vi "val_vagy_vel.vi"(11 "Becenév":string) -> (3 "-val/vel rag":waveform(dbl)[](array[waveform]))   [LabVIEW 2014]
panel:
  out "Boolean":bool
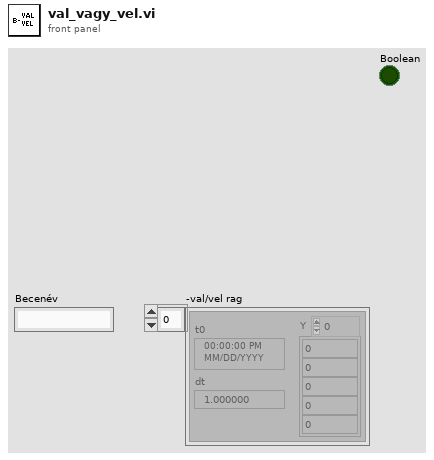
[diagram p1: front panel]
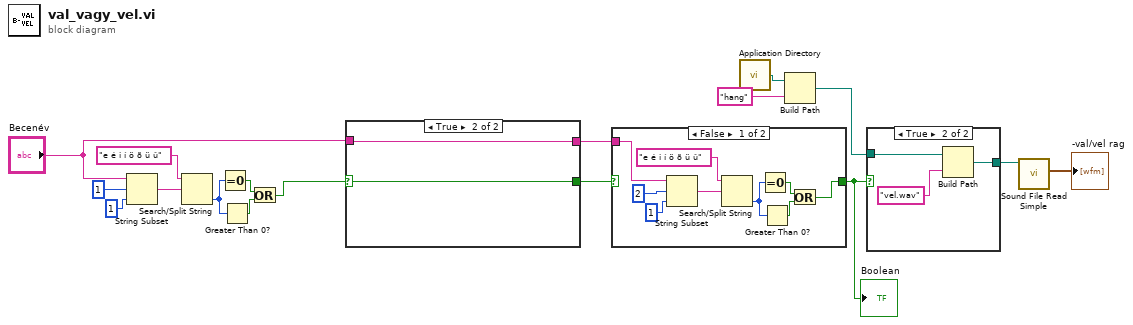
[diagram p0: block diagram]
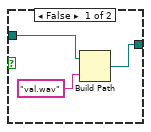
[diagram p2: hidden frame]
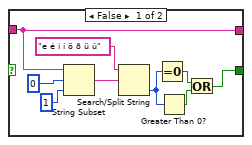
[diagram p4: hidden frame]
diagram:
  n1 = String Subset(string="Becenév", offset (0)=1, length (rest)=1 ("length (rest)")) -> (substring=w10:string)
  n2 = Search/Split String(string="e é i í ö õ ü û" ("search string/char (-)"), search string/char (-)=w10) -> (offset of match=w9:i32)  [unwired: 1 in, 2 out]
  n3 = Equal To 0?(x=w9) -> (x = 0?=w13:bool)
  n4 = Greater Than 0?(x=w9) -> (x > 0?=w14:bool)
  n5 = Or(x=w13, y=w14) -> (x .or. y?=w16:bool)
  n6 = case shown="True" w16 {
    selector: w16 -> [_ w28]
    tunnel: [w19 w28] -> w8
    tunnel: "Becenév" -> [w18 w27]
    tunnel: [w18 w27] -> w1
    frame False {
      n7 = String Subset(string=w18, offset (0)=0, length (rest)=1 ("length (rest)")) -> (substring=w25:string)
      n8 = Search/Split String(string="e é i í ö õ ü û" ("search string/char (-)"), search string/char (-)=w25) -> (offset of match=w26:i32)  [unwired: 1 in, 2 out]
      n9 = Equal To 0?(x=w26) -> (x = 0?=w22:bool)
      n10 = Greater Than 0?(x=w26) -> (x > 0?=w21:bool)
      n11 = Or(x=w22, y=w21) -> (x .or. y?=w19:bool)
    }
    frame True {
    }
  }
  n12 = case shown="False" w8 {
    selector: w8 -> [_ w38]
    tunnel: [w30 w38] -> w3
    tunnel: w1 -> [w29 _]
    frame False {
      n13 = String Subset(string=w29, offset (0)=2, length (rest)=1 ("length (rest)")) -> (substring=w36:string)
      n14 = Search/Split String(string="e é i í ö õ ü û" ("search string/char (-)"), search string/char (-)=w36) -> (offset of match=w37:i32)  [unwired: 1 in, 2 out]
      n15 = Equal To 0?(x=w37) -> (x = 0?=w33:bool)
      n16 = Greater Than 0?(x=w37) -> (x > 0?=w32:bool)
      n17 = Or(x=w33, y=w32) -> (x .or. y?=w30:bool)
    }
    frame True {
    }
  }
  "Boolean" <- w3
  n18 = call <vilib>:"Application Directory.vi"() -> ("Application Directory"=w7:path)
  n19 = Build Path(base path=w7, name or relative path="hang") -> (appended path=w6:path)
  n20 = case shown="True" w3 {
    tunnel: w6 -> [w40 w43]
    tunnel: [w39 w42] -> w5
    frame False {
      n21 = Build Path(base path=w40, name or relative path="val.wav") -> (appended path=w39:path)
    }
    frame True {
      n22 = Build Path(base path=w43, name or relative path="vel.wav") -> (appended path=w42:path)
    }
  }
  n23 = call <vilib>:"Sound File Read Simple.vi"("path"=w5) -> ("data"=→"-val/vel rag":waveform(dbl)[])  [unwired: 7 in, 3 out]
